vi "DAQ1.vi"(6 "sampling info":cluster{"Fs":dbl, "#s":dbl}={"Fs"=10000.0, "#s"=1000.0}) -> (0 "Waveform":waveform(dbl)={"t0"=timestamp(42.1 s since 1904-01-01), "dt"=0.0001, "Y"=array[1000 elements]})   [LabVIEW 2018]
uses:
  <vilib>/measure/NI_MABase.lvlib
panel:
  in  "phase":dbl=45.0 format="%.2p"
  in  "rumore":dbl=0.02 min=0.0 step=0.01 format="%.2p"
  in  "signal type":T1(ring)
  in  "amplitude":dbl=3.0 format="%0.2p"
  in  "frequency":dbl=50.0 min=0.0 step=0.5 format="%0.2p"
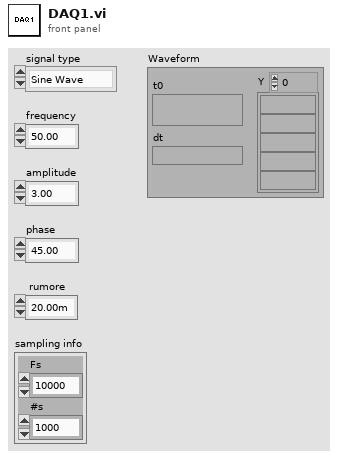
[diagram p1: front panel]
types:
  T1 = enum16{"Sine Wave", "Triangle Wave", "Square Wave", "Sawtooth Wave"}
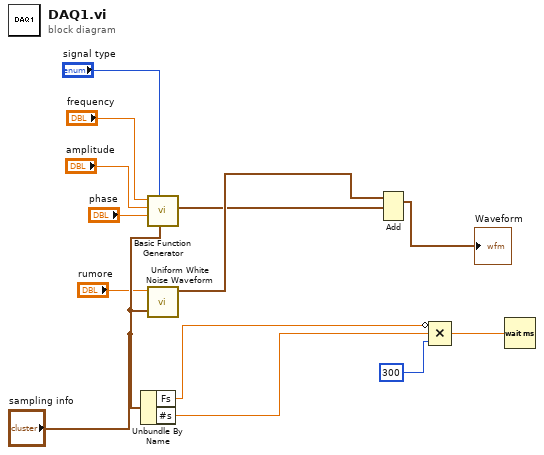
[diagram p0: block diagram]
diagram:
  n1 = Unbundle By Name("sampling info") -> ("Fs"=w5:dbl, "#s"=w6:dbl)
  n2 = call <vilib>:"Basic Function Generator.vi"("sampling info"="sampling info", "signal type"="signal type", "phase"="phase", "amplitude"="amplitude", "frequency"="frequency") -> ("signal out"=w10:waveform(dbl))  [unwired: 4 in, 2 out]
  n3 = call <vilib>:"Uniform White Noise Waveform.vi"("sampling info"="sampling info", "amplitude"="rumore") -> ("signal out"=w11:waveform(dbl))  [unwired: 8 in, 1 out]
  n4 = Add(1:w10, 2:w11) -> (0:→"Waveform":waveform(dbl))  [unwired: 1 in, 1 out]
  n5 = Compound Arithmetic op=MULTIPLY(invert w5, w6, u32 300 ("millisecond timer value")) -> (w8:dbl)
  n6 = Wait (ms)(milliseconds to wait=w8) -> ()  [unwired: 1 out]
